vi "New Log File Configuration.vi"(8 "error in (no error)":errorcluster, 9 "Default Log Directory":string[](array[string]), 10 "Default Name":string="Log File", 11 "Device Ref in":T1=18446744073709551615 format="%.0x") -> (0 "error out":errorcluster, 3 "Device Ref out":T1 format="%.0x")   [LabVIEW 2018, in "Embedded Data Logger System Explorer.lvlib"]
uses:
  Embedded Data Logger System Explorer.lvlib
  <vilib>/NI Veristand/Custom Device API/Custom Device Item Ref.ctl
  <vilib>/NI Veristand/Custom Device API/Custom Device Channel.ctl
  <vilib>/NI Veristand/Custom Device API/Custom Device Channel Type.ctl
  Shared/Constants.vi
  <vilib>/NI Veristand/Custom Device API/Set Item Property (String Array).vi
  <vilib>/NI Veristand/Custom Device API/Set Item Property (Boolean).vi
  <vilib>/NI Veristand/Custom Device API/Custom Device API.lvlib
  Shared/Embedded Data Logger Shared.lvlib
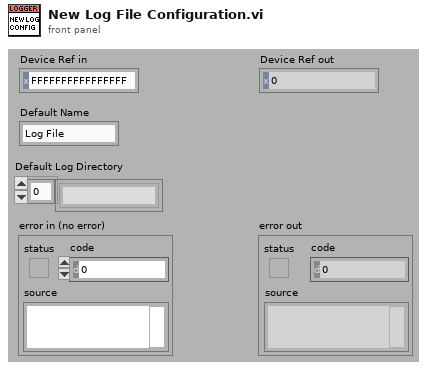
[diagram p1: front panel]
types:
  T1 = typedef "Custom Device API.lvlib/Custom Device Item Ref.ctl" = u64
  T2 = typedef "Custom Device API.lvlib/Custom Device Channel Type.ctl" = enum16{"Input", "Output"}
  T3 = typedef "Custom Device API.lvlib/Custom Device Channel.ctl" = cluster{"Type":T2, "Units":string, "Default Value":dbl, "Faultable":bool, "Scalable":bool}
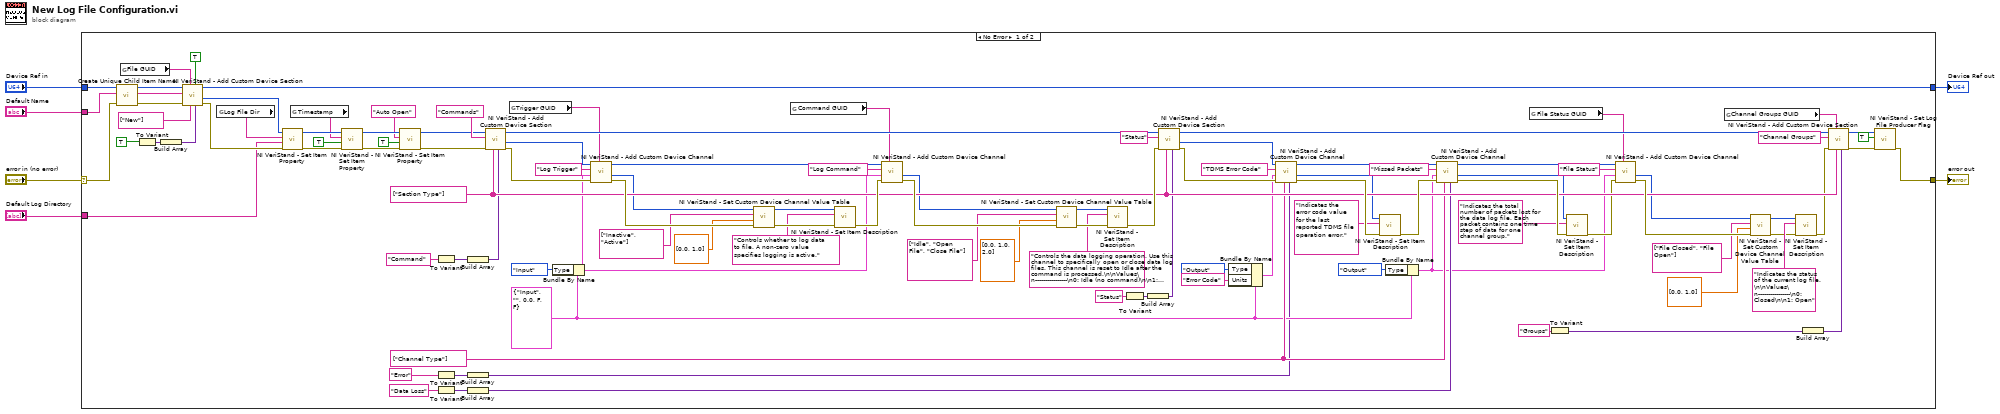
[diagram p0: block diagram]
diagram:
  n1 = case shown="No Error" "error in (no error)" {
    selector: "error in (no error)" -> [w69 w116]
    tunnel: "Default Name" -> [w99 _]
    tunnel: "Default Log Directory" -> [w9 _]
    tunnel: "Device Ref in" -> [w90 w117]
    tunnel: [w89 w117] -> w3
    tunnel: [w25 w116] -> w2
    frame No Error {
      w101 = string[] ["Channel Type"] ("Property names")
      w63 = T3 {"Type"=enum."Input", "Units"="", "Default Value"=0.0, "Faultable"=FALSE, "Scalable"=FALSE} ("Channel")
      w102 = string[] ["Section Type"] ("Property names")
      n2 = call "Create Unique Child Item Name.vi"("error in (no error)"=w69, "Name in"=w99, "Parent Item Ref in"=w90) -> ("error out"=w98:errorcluster, "Unique Name out"=w96:string, "Parent Item Ref out"=w97:T1)  [unwired: 6 out]
      n3 = global read "Constants.vi" "File GUID"() -> (w14:string)
      n4 = To Variant(anything=TRUE) -> (Variant=w46:variant)
      n5 = Build Array(w46) -> (w45:variant[])
      n6 = call <vilib>:"NI VeriStand - Add Custom Device Section.vi"("Property Values"=w45, "Highlight? (F)"=TRUE, "Property names"=string[] ["New"], "GUID (Default Section)"=w14, "error in (no error)"=w98, "Section Name"=w96, "Parent Ref in"=w97) -> ("error out"=w100:errorcluster, "Section Ptr"=w91:T1, "Parent Ref out"=w89:T1)  [unwired: 2 out]
      n7 = global read "Constants.vi" "Log File Dir"() -> (w8:string)
      n8 = call-poly <vilib>:"NI VeriStand - Set Item Property.vi"("error in (no error)"=w100, "Value"=w9, "Property Name"=w8, "Item Ref in"=w91) -> ("error out"=w94:errorcluster, "Item Ref out"=w95:T1)  [unwired: 6 out]
      n9 = global read "Constants.vi" "Timestamp"() -> (w7:string)
      n10 = call-poly <vilib>:"NI VeriStand - Set Item Property.vi"("error in (no error)"=w94, "Value"=TRUE, "Property Name"=w7, "Item Ref in"=w95) -> ("error out"=w36:errorcluster, "Item Ref out"=w40:T1)  [unwired: 6 out]
      n11 = call-poly <vilib>:"NI VeriStand - Set Item Property.vi"("error in (no error)"=w36, "Value"=TRUE, "Property Name"="Auto Open", "Item Ref in"=w40) -> ("error out"=w37:errorcluster, "Item Ref out"=w38:T1)  [unwired: 6 out]
      n12 = To Variant(anything="Command" ("String")) -> (Variant=w87:variant)
      n13 = To Variant(anything="Error" ("String")) -> (Variant=w67:variant)
      n14 = To Variant(anything="Data Loss" ("String")) -> (Variant=w62:variant)
      n15 = Build Array(w87) -> (w88:variant[])
      n16 = Build Array(w67) -> (w59:variant[])
      n17 = Build Array(w62) -> (w60:variant[])
      n18 = call <vilib>:"NI VeriStand - Add Custom Device Section.vi"("Property Values"=w88, "Property names"=w102, "error in (no error)"=w37, "Section Name"="Commands", "Parent Ref in"=w38) -> ("error out"=w84:errorcluster, "Section Ptr"=w85:T1, "Parent Ref out"=w80:T1)  [unwired: 2 in, 2 out]
      n19 = global read "Constants.vi" "Trigger GUID"() -> (w13:string)
      n20 = Bundle By Name(cluster=w63, "Type"=Custom_Device_Channel_Type."Input") -> (w42:T3)
      n21 = call <vilib>:"NI VeriStand - Add Custom Device Channel.vi"("GUID (Default Channel)"=w13, "error in (no error)"=w84, "Channel"=w42, "Channel Name"="Log Trigger", "Parent Ref in"=w85) -> ("error out"=w113:errorcluster, "Channel Ref"=w20:T1, "Parent Ref out"=w43:T1)  [unwired: 3 in, 1 out]
      n22 = call <vilib>:"NI VeriStand - Set Custom Device Channel Value Table.vi"("error in (no error)"=w113, "Values"=dbl[] [0.0, 1.0], "Names"=string[] ["Inactive", "Active"], "Channel Ref in"=w20) -> ("error out"=w109:errorcluster, "Channel Ref out"=w21:T1)  [unwired: 6 in]
      n23 = global read "Constants.vi" "Command GUID"() -> (w12:string)
      n24 = call <vilib>:"NI VeriStand - Set Item Description.vi"("error in (no error)"=w109, "Description"="Controls whether to log data to file. A non-zero value specifies logging is active." ("String"), "Item Ref in"=w21) -> ("error out"=w107:errorcluster)  [unwired: 6 in, 2 out]
      n25 = call <vilib>:"NI VeriStand - Add Custom Device Channel.vi"("GUID (Default Channel)"=w12, "error in (no error)"=w107, "Channel"=w42, "Channel Name"="Log Command", "Parent Ref in"=w43) -> ("error out"=w114:errorcluster, "Channel Ref"=w24:T1)  [unwired: 3 in, 2 out]
      n26 = call <vilib>:"NI VeriStand - Set Custom Device Channel Value Table.vi"("error in (no error)"=w114, "Values"=dbl[] [0.0, 1.0, 2.0], "Names"=string[] ["Idle", "Open File", "Close File"], "Channel Ref in"=w24) -> ("error out"=w108:errorcluster, "Channel Ref out"=w23:T1)  [unwired: 6 in]
      n27 = call <vilib>:"NI VeriStand - Set Item Description.vi"("error in (no error)"=w108, "Description"="Controls the data logging operation. Use this channel to specifically open or close data log files. This channel is reset to Idle after the command is processed.\n\nValues\n----------------\n0: Idle (no command)\n\n1: Open File. Closes the previous file reference if it was open and opens a new file reference.\n\n2: Close File. Closes the file reference without opening a new file reference." ("String"), "Item Ref in"=w23) -> ("error out"=w106:errorcluster)  [unwired: 6 in, 2 out]
      n28 = To Variant(anything="Status" ("String")) -> (Variant=w79:variant)
      n29 = Build Array(w79) -> (w78:variant[])
      n30 = call <vilib>:"NI VeriStand - Add Custom Device Section.vi"("Property Values"=w78, "Property names"=w102, "error in (no error)"=w106, "Section Name"="Status", "Parent Ref in"=w80) -> ("error out"=w75:errorcluster, "Section Ptr"=w76:T1, "Parent Ref out"=w58:T1)  [unwired: 2 in, 2 out]
      n31 = Bundle By Name(cluster=w63, "Type"=Custom_Device_Channel_Type."Output", "Units"="Error Code") -> (w72:T3)
      n32 = call <vilib>:"NI VeriStand - Add Custom Device Channel.vi"("Property Values"=w59, "Property names"=w101, "error in (no error)"=w75, "Channel"=w72, "Channel Name"="TDMS Error Code", "Parent Ref in"=w76) -> ("error out"=w105:errorcluster, "Channel Ref"=w52:T1, "Parent Ref out"=w66:T1)  [unwired: 2 in, 1 out]
      n33 = call <vilib>:"NI VeriStand - Set Item Description.vi"("error in (no error)"=w105, "Description"="Indicates the error code value for the last reported TDMS file operation error." ("String"), "Item Ref in"=w52) -> ("error out"=w103:errorcluster)  [unwired: 6 in, 2 out]
      n34 = Bundle By Name(cluster=w63, "Type"=Custom_Device_Channel_Type."Output") -> (w31:T3)
      n35 = call <vilib>:"NI VeriStand - Add Custom Device Channel.vi"("Property Values"=w60, "Property names"=w101, "error in (no error)"=w103, "Channel"=w31, "Channel Name"="Missed Packets", "Parent Ref in"=w66) -> ("error out"=w104:errorcluster, "Channel Ref"=w50:T1, "Parent Ref out"=w33:T1)  [unwired: 2 in, 1 out]
      n36 = global read "Constants.vi" "File Status GUID"() -> (w11:string)
      n37 = To Variant(anything="Groups" ("String")) -> (Variant=w55:variant)
      n38 = call <vilib>:"NI VeriStand - Set Item Description.vi"("error in (no error)"=w104, "Description"="Indicates the total number of packets lost for the data log file. Each packet contains one time step of data for one channel group." ("String"), "Item Ref in"=w50) -> ("error out"=w32:errorcluster)  [unwired: 6 in, 2 out]
      n39 = call <vilib>:"NI VeriStand - Add Custom Device Channel.vi"("GUID (Default Channel)"=w11, "error in (no error)"=w32, "Channel"=w31, "Channel Name"="File Status", "Parent Ref in"=w33) -> ("error out"=w115:errorcluster, "Channel Ref"=w16:T1)  [unwired: 3 in, 2 out]
      n40 = global read "Constants.vi" "Channel Groups GUID"() -> (w10:string)
      n41 = call <vilib>:"NI VeriStand - Set Custom Device Channel Value Table.vi"("error in (no error)"=w115, "Values"=dbl[] [0.0, 1.0], "Names"=string[] ["File Closed", "File Open"], "Channel Ref in"=w16) -> ("error out"=w18:errorcluster, "Channel Ref out"=w17:T1)  [unwired: 6 in]
      n42 = call <vilib>:"NI VeriStand - Set Item Description.vi"("error in (no error)"=w18, "Description"="Indicates the status of the current log file.\n\nValues\n----------------\n0: Closed\n\n1: Open" ("String"), "Item Ref in"=w17) -> ("error out"=w29:errorcluster)  [unwired: 6 in, 2 out]
      n43 = Build Array(w55) -> (w54:variant[])
      n44 = call <vilib>:"NI VeriStand - Add Custom Device Section.vi"("Property Values"=w54, "Property names"=w102, "GUID (Default Section)"=w10, "error in (no error)"=w29, "Section Name"="Channel Groups", "Parent Ref in"=w58) -> ("error out"=w27:errorcluster, "Parent Ref out"=w28:T1)  [unwired: 1 in, 3 out]
      n45 = call <vilib>:"NI VeriStand - Set Log File Producer Flag.vi"("error in (no error)"=w27, "Log File Producer"=TRUE ("Log File Provider"), "Item Ref in"=w28) -> ("error out"=w25:errorcluster)  [unwired: 7 in, 1 out]
    }
    frame Error {
    }
  }
  "Device Ref out" <- w3
  "error out" <- w2
